vi "FT OPEN SENCILLO.vi"(0 "CTA Test#":string) -> (1 "States":T1, 2 "Handle":u32)   [LabVIEW 2009]
uses:
  Machine State.ctl
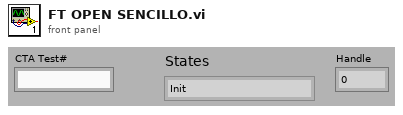
[diagram p1: front panel]
types:
  T1 = typedef "Machine State.ctl" = enum16{"Init", "Config Test", "Power Start", "Ft232 Start", "Seleccion Vasic", "Test Registros", "Test ADC Inicial", "Test ADC", "Test Func Transferencia", "Test Func Transferencia Sumadores", "Test Offset Analogico", "Test Offset Digital", "Loop Vasic", "Generate Report", "Ft232 Stop", "Power Stop", "Exit", "Error"}
  T2 = cluster{"Device Index":u32, "FT_FLAGS_OPENED":bool, "FT_FLAGS_HISPEED":bool, "Type":u32, "VID":u32, "PID":u32, "LocID":i32, "Serial Number":string, "Description":string, "FT_Handle":u32}[]
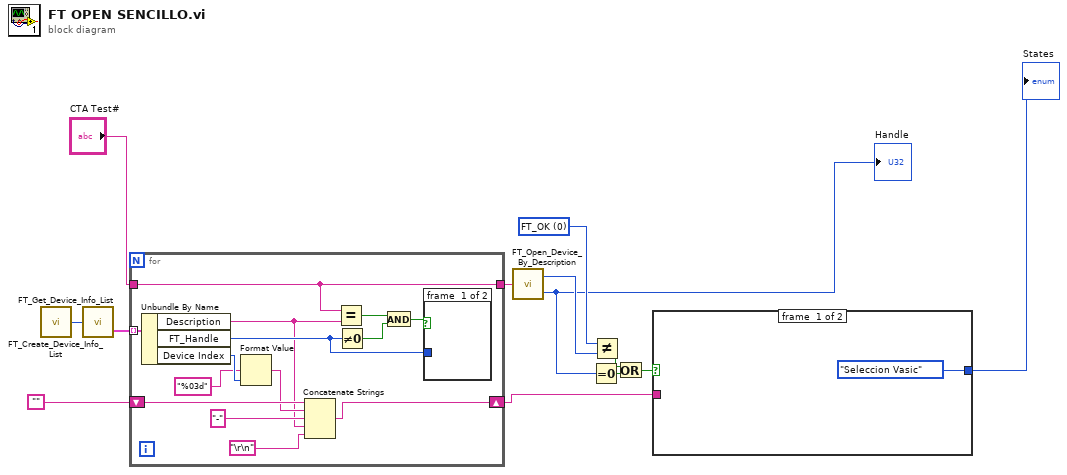
[diagram p0: block diagram]
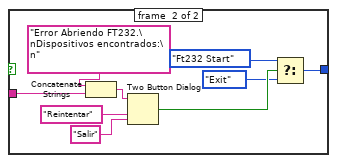
[diagram p2: hidden frame]
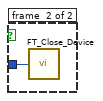
[diagram p3: hidden frame]
diagram:
  w9 = u32 0 items=["FT_OK", "FT_INVALID_HANDLE", "FT_DEVICE_NOT_FOUND", "FT_DEVICE_NOT_OPENED", "FT_IO_ERROR", "FT_INSUFFICIENT_RESOURCES", "FT_INVALID_PARAMETER", "FT_INVALID_BAUD_RATE", "FT_DEVICE_NOT_OPENED_FOR_ERASE", "FT_DEVICE_NOT_OPENED_FOR_WRITE", "FT_FAILED_TO_WRITE_DEVICE", "FT_EEPROM_READ_FAILED", "FT_EEPROM_WRITE_FAILED", "FT_EEPROM_ERASE_FAILED", "FT_EEPROM_NOT_PRESENT", "FT_EEPROM_NOT_PROGRAMMED", "FT_INVALID_ARGS", "FT_NOT_SUPPORTED", "FT_OTHER_ERROR"] ("FT_Status")
  n1 = call "FT_Create_Device_Info_List.vi"() -> ("Number of Devices"=w1:u32)  [unwired: 1 out]
  n2 = call "FT_Get_Device_Info_List.vi"("Number Of Devices"=w1) -> ("Device Info List"=w2:T2)  [unwired: 1 out]
  n3 = for {
    tunnel: w2 -> [w27] mode=indexing
    tunnel: "CTA Test#" -> [w26]
    tunnel: [w26] -> w4
    shift-right: [w20] -> w13
    shift-left: "" -> [w21]
    n4 = Unbundle By Name(w27) -> ("Description"=w15:string, "FT_Handle"=w22:u32, "Device Index"=w19:u32)
    n5 = Format Value(format string="%03d", value (0)=w19) -> (output string=w17:string)  [unwired: 1 in]
    n6 = Concatenate Strings(w21, w17, "-" ("string"), w15, "\r\n") -> (w20:string)
    n7 = Equal?(x=w26, y=w15) -> (x = y?=w24:bool)
    n8 = Not Equal To 0?(x=w22) -> (x != 0?=w25:bool)
    n9 = And(x=w24, y=w25) -> (x .and. y?=w23:bool)
    n10 = case shown="False" w23 {
      tunnel: w22 -> [_ w28]
      frame #0 {
      }
      frame #1 {
        n11 = call "FT_Close_Device.vi"("Handle"=w28) -> ()  [unwired: 1 out]
      }
    }
  }
  n12 = call "FT_Open_Device_By_Description.vi"("Device Description"=w4) -> ("FT_Status"=w8:u32, "Handle"=w5:u32)
  "Handle" <- w5
  n13 = Equal To 0?(x=w5) -> (x = 0?=w6:bool)
  n14 = Not Equal?(x=w9, y=w8) -> (x != y?=w7:bool)
  n15 = Or(x=w7, y=w6) -> (x .or. y?=w10:bool)
  n16 = case shown="True" w10 {
    tunnel: [Machine_State."Seleccion Vasic" ("States") w33] -> w11
    tunnel: w13 -> [_ w30]
    frame #0 {
    }
    frame #1 {
      n17 = Concatenate Strings("Error Abriendo FT232.\nDispositivos encontrados:\n" ("message"), w30) -> (w31:string)
      n18 = Two Button Dialog(message=w31, 1:"Salir" ("F button name (\"Cancel\")"), 2:"Reintentar" ("T button name (\"OK\")")) -> (T button?=w36:bool)
      n19 = Select(t=Machine_State."Ft232 Start" ("States"), s=w36, f=Machine_State."Exit" ("States")) -> (s? t:f=w33:T1)
    }
  }
  "States" <- w11
